vi "LINC COSMOS Update Item.vi"(4 "property":T1(ring), 5 "ignore":bool, 6 "item":T2, 7 "macro":T3, 8 "error in (no error)":errorcluster, 9 "item index":i32, 10 "packet index":i32, 11 "packets in":T4[](array[typedef])) -> (0 "error out":errorcluster, 3 "packets out":T4[](array[typedef]))   [LabVIEW 2018, in "STEPkgDriver_LINC.lvlib"]
uses:
  STEPkgDriver_LINC.lvlib
  LINC Format Prototype.ctl
  LINC Packet.ctl
  LINC Macro.ctl
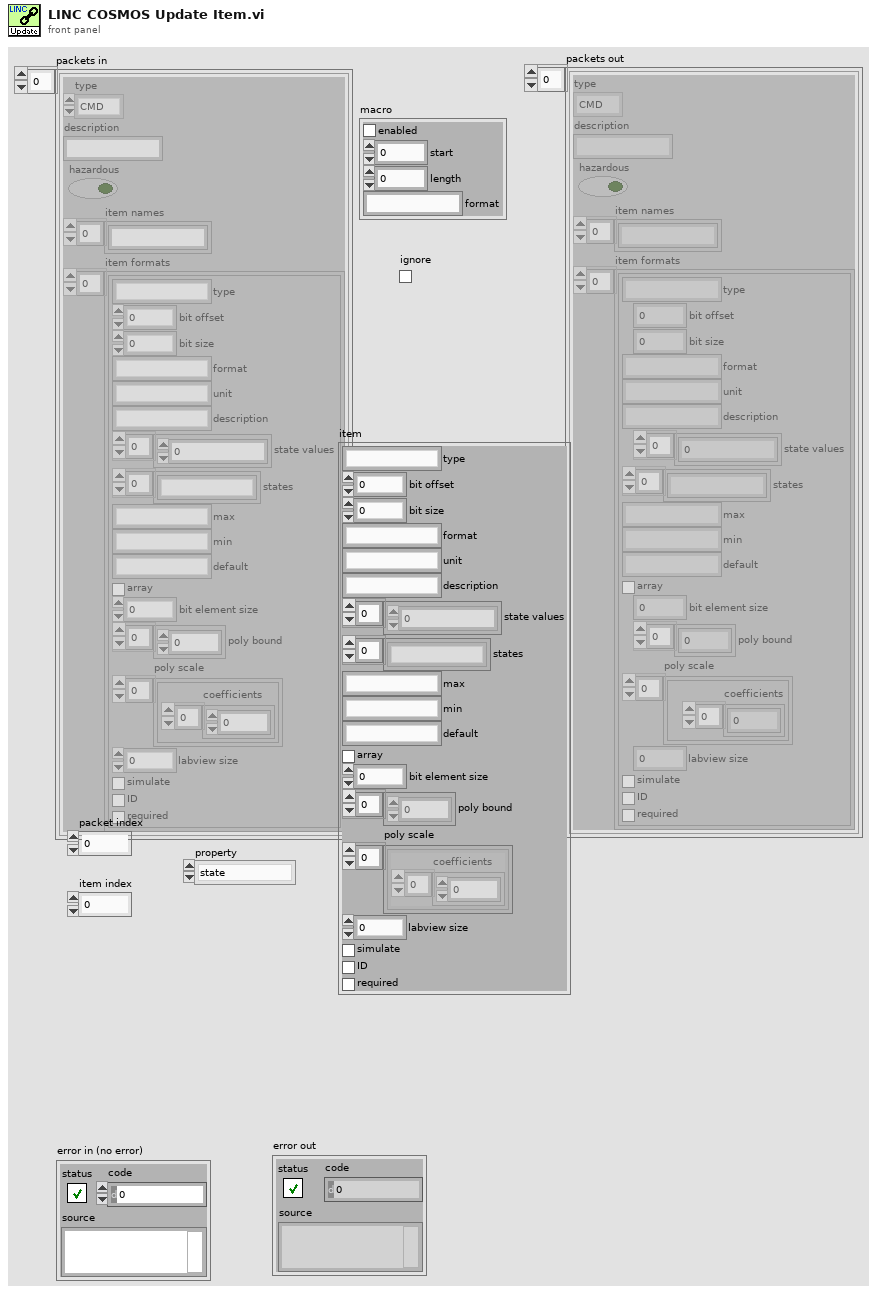
[diagram p1: front panel]
types:
  T1 = enum16{"state", "required", "poly scale", "format string", "minimum value", "maximum value", "default value", "description", "units"}
  T2 = typedef "STEPkgDriver_LINC.lvlib/LINC Format Prototype.ctl" = cluster{"type":string, "bit offset":i32, "bit size":i32, "format":string, "unit":string, "description":string, "state values":i64[], "states":string[], "max":string, "min":string, "default":string, "array":bool, "bit element size":i32, "poly bound":dbl[], "poly scale":cluster{"coefficients":dbl[]}[], "labview size":i32, "simulate":bool, "ID":bool, "required":bool}
  T3 = typedef "STEPkgDriver_LINC.lvlib/LINC Macro.ctl" = cluster{"enabled":bool, "start":i32, "length":i32, "format":string}
  T4 = typedef "STEPkgDriver_LINC.lvlib/LINC Packet.ctl" = cluster{"type":enum16{"CMD", "TLM"}, "description":string, "hazardous":bool, "item names":string[], "item formats":T2[]}
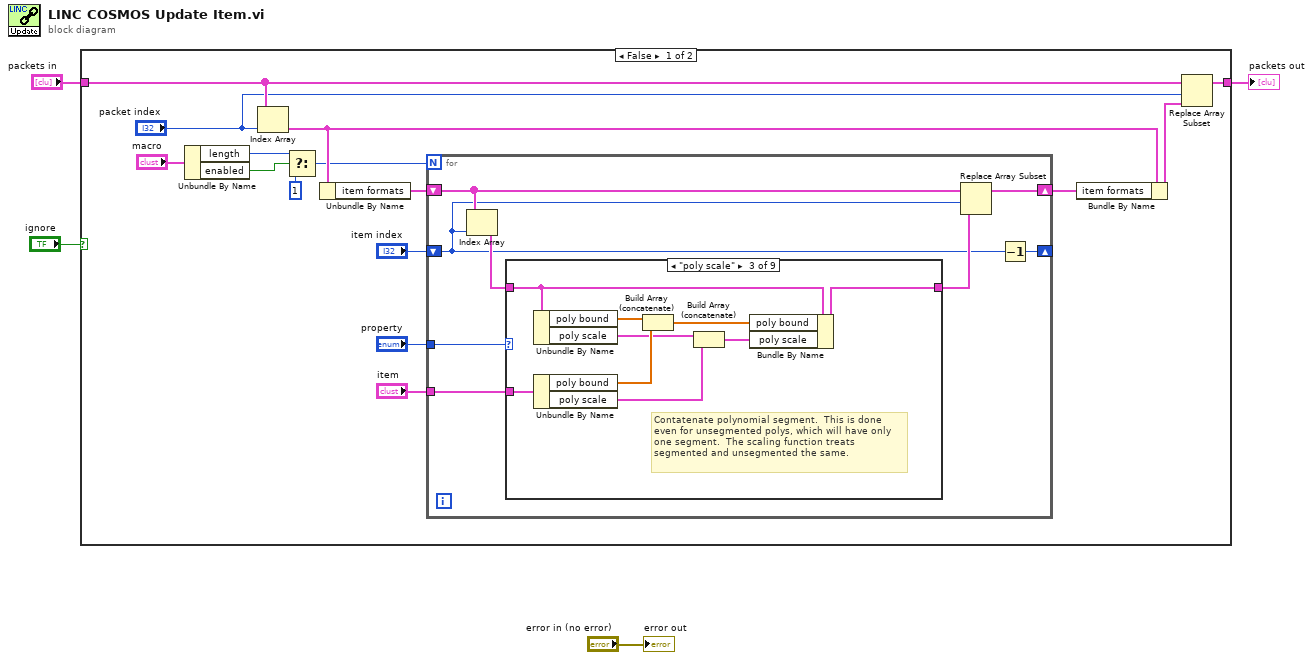
[diagram p0: block diagram]
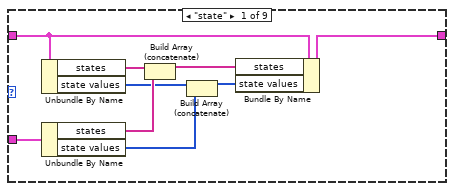
[diagram p2: hidden frame]
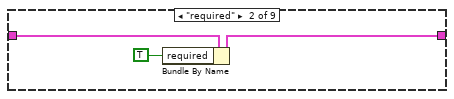
[diagram p3: hidden frame]
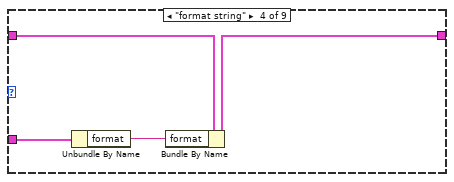
[diagram p4: hidden frame]
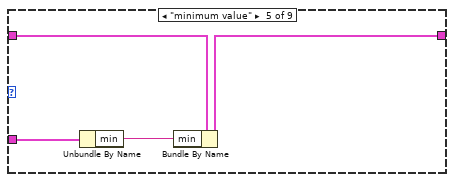
[diagram p5: hidden frame]
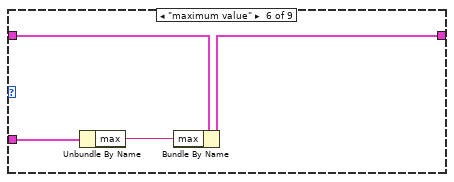
[diagram p6: hidden frame]
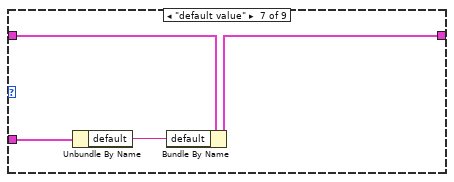
[diagram p7: hidden frame]
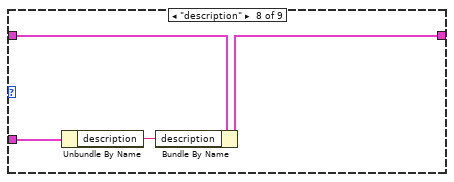
[diagram p8: hidden frame]
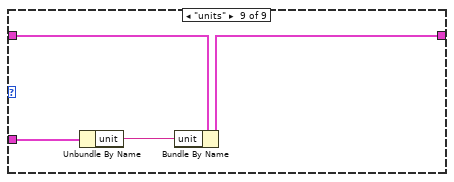
[diagram p9: hidden frame]
diagram:
  n1 = case shown="False" "ignore" {
    tunnel: "packets in" -> [w19 w73]
    tunnel: [w18 w73] -> w3
    frame False {
      n2 = Unbundle By Name("macro") -> ("length"=w13:i32, "enabled"=w14:bool)
      n3 = Index Array(array=w19, index="packet index") -> (element=w9:T4)
      n4 = Select(t=w13, s=w14, f=1) -> (s? t:f=w7:i32)
      n5 = Unbundle By Name(w9) -> ("item formats"=w11:T2[])
      n6 = for {
        N: w7 -> [_]
        shift-right: [w24] -> w12
        shift-left: w11 -> [w25]
        shift-right: [w22] -> _
        shift-left: "item index" -> [w23]
        tunnel: "item" -> [w21]
        tunnel: "property" -> [w20]
        n7 = Index Array(array=w25, index=w23) -> (element=w27:T2)
        n8 = case shown="\"poly scale\"" w20 {
          tunnel: w27 -> [w34 w39 w46 w52 w56 w60 w64 w68 w72]
          tunnel: [w36 w38 w48 w51 w55 w59 w63 w67 w71] -> w26
          tunnel: w21 -> [w35 _ w47 w50 w54 w58 w62 w66 w70]
          frame "state" {
            n9 = Unbundle By Name(w34) -> ("states"=w33:string[], "state values"=w30:i64[])
            n10 = Unbundle By Name(w35) -> ("states"=w31:string[], "state values"=w28:i64[])
            n11 = Build Array (concatenate)(w33, w31) -> (w32:string[])
            n12 = Build Array (concatenate)(w30, w28) -> (w29:i64[])
            n13 = Bundle By Name(cluster=w34, "states"=w32, "state values"=w29) -> (w36:T2)
          }
          frame "required" {
            n14 = Bundle By Name(cluster=w39, "required"=TRUE ("REQUIRED")) -> (w38:T2)
          }
          frame "poly scale" {
            # "Contatenate polynomial segment.  This is done even for unsegmented polys, which will have only one segment.  The scaling function treats segmented and unsegmented the same."
            n15 = Unbundle By Name(w46) -> ("poly bound"=w45:dbl[], "poly scale"=w42:cluster{"coefficients":dbl[]}[])
            n16 = Unbundle By Name(w47) -> ("poly bound"=w44:dbl[], "poly scale"=w41:cluster{"coefficients":dbl[]}[])
            n17 = Build Array (concatenate)(w45, w44) -> (w43:dbl[])
            n18 = Build Array (concatenate)(w42, w41) -> (w40:cluster{"coefficients":dbl[]}[])
            n19 = Bundle By Name(cluster=w46, "poly bound"=w43, "poly scale"=w40) -> (w48:T2)
          }
          frame "format string" {
            n20 = Unbundle By Name(w50) -> ("format"=w49:string)
            n21 = Bundle By Name(cluster=w52, "format"=w49) -> (w51:T2)
          }
          frame "minimum value" {
            n22 = Unbundle By Name(w54) -> ("min"=w53:string)
            n23 = Bundle By Name(cluster=w56, "min"=w53) -> (w55:T2)
          }
          frame "maximum value" {
            n24 = Unbundle By Name(w58) -> ("max"=w57:string)
            n25 = Bundle By Name(cluster=w60, "max"=w57) -> (w59:T2)
          }
          frame "default value" {
            n26 = Unbundle By Name(w62) -> ("default"=w61:string)
            n27 = Bundle By Name(cluster=w64, "default"=w61) -> (w63:T2)
          }
          frame "description" {
            n28 = Unbundle By Name(w66) -> ("description"=w65:string)
            n29 = Bundle By Name(cluster=w68, "description"=w65) -> (w67:T2)
          }
          frame "units" {
            n30 = Unbundle By Name(w70) -> ("unit"=w69:string)
            n31 = Bundle By Name(cluster=w72, "unit"=w69) -> (w71:T2)
          }
        }
        n32 = Replace Array Subset(array=w25, new element=w26, index=w23) -> (w24:T2[])
        n33 = Decrement(x=w23) -> (x-1=w22:i32)
      }
      n34 = Bundle By Name(cluster=w9, "item formats"=w12) -> (w10:T4)
      n35 = Replace Array Subset(array=w19, new element=w10, index="packet index") -> (w18:T4[])
    }
    frame True {
    }
  }
  "packets out" <- w3
  "error out" <- "error in (no error)"
